vi "MenuButtons.vi"() -> ()   [LabVIEW 2023]
panel:
  in  "ME":bool
  in  "Tacho Interface":bool
  in  "IO Interface":bool
  in  "Datalogger":bool
  in  "Control Station 2":bool
  in  "SF lgi mK1.2 2":bool
  in  "RCS Status":bool
  in  "Cylinder Lubrication":bool
  in  "Shaft Generator":bool
  in  "Axial Vibration":bool
  in  "Hydraulic Power Supply":bool
  in  "Safety System":bool
  in  "Auxiliary System":bool
  in  "Cylinder Configuration":bool
  in  "Turbocharger":bool
  in  "Long Term Test":bool
  in  "Testwall Status":bool
  in  "Report Issue":bool
  in  "Controller Interface":bool
  in  "User Utils":bool
  in  "About":bool
  in  "MOP Parameters":bool
  in  "Update to latest version":bool
  in  "Super Restart Simulation":bool
  in  "MQTT Subscriber":bool
  in  "Show Context Help":bool
  in  "Show Block Diagram":bool
  in  "LabVIEWDev":bool
  in  "Signals On Engine":bool
  in  "Control Station":bool
  in  "Restart Simulation":bool
  in  "Close Screen":bool
  in  "Operate":bool
  # "There's a few of these!"
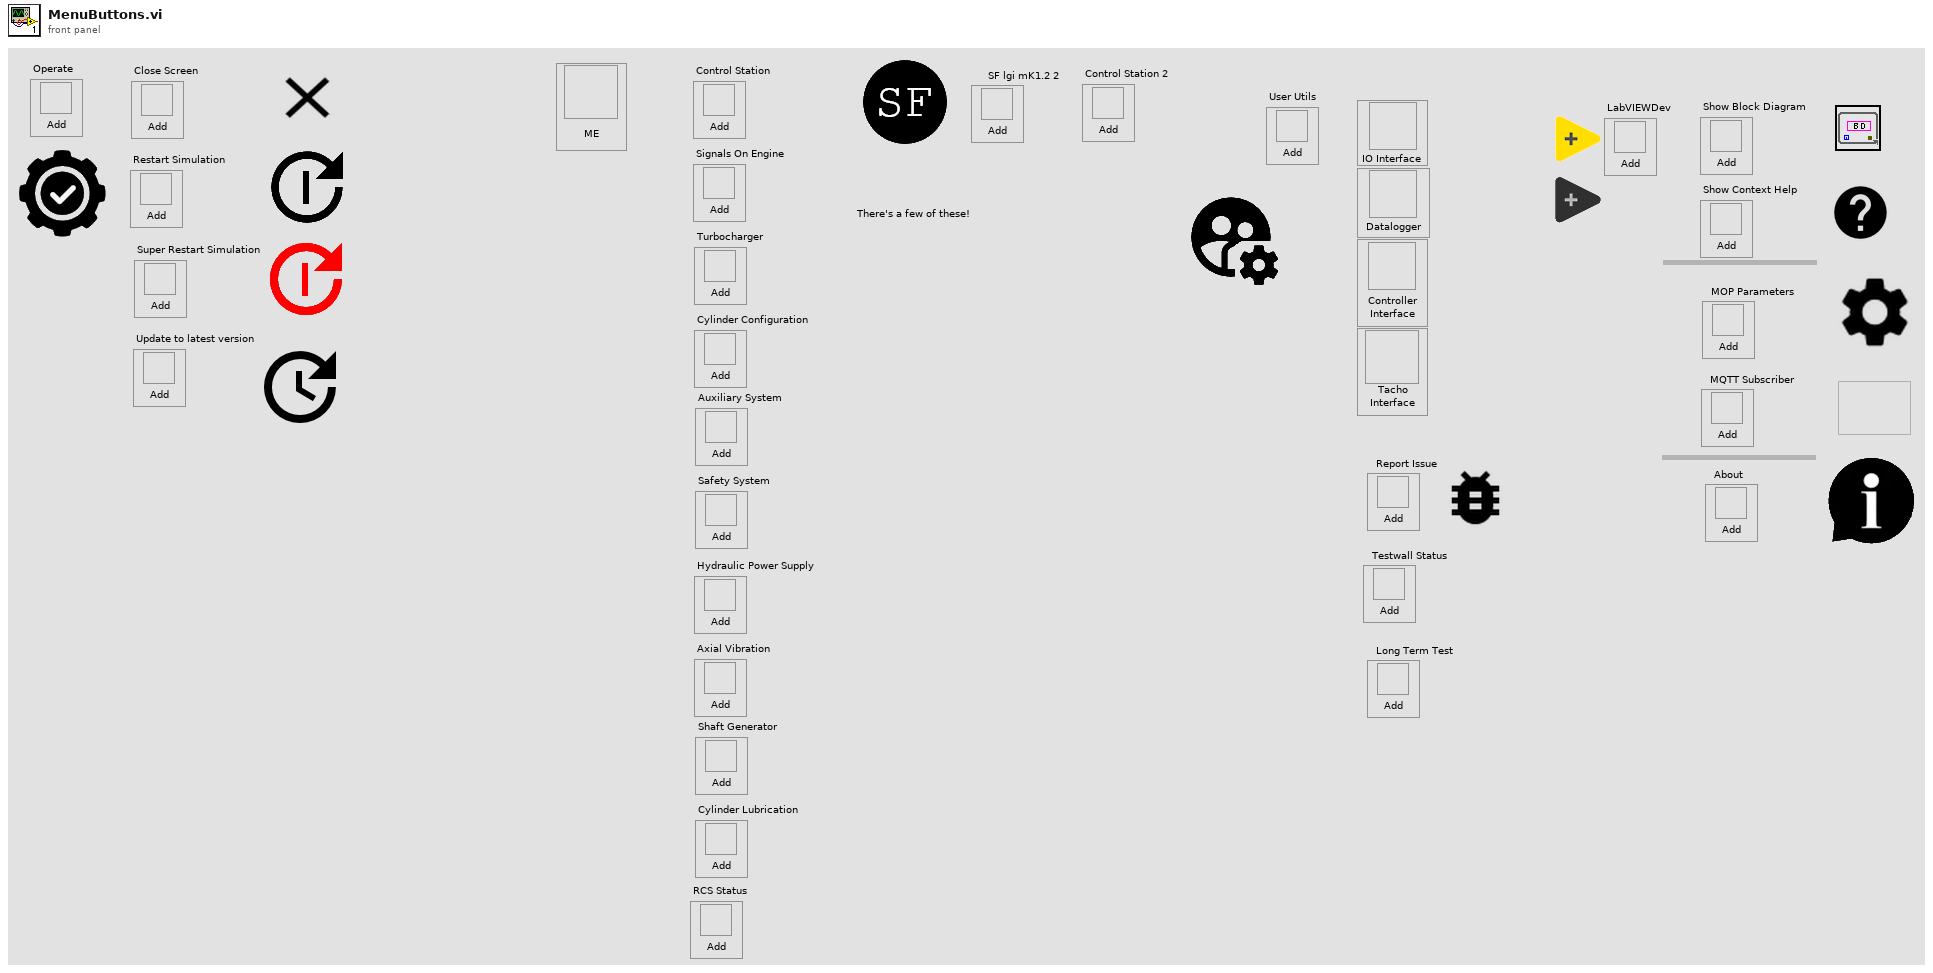
[diagram p1: front panel]
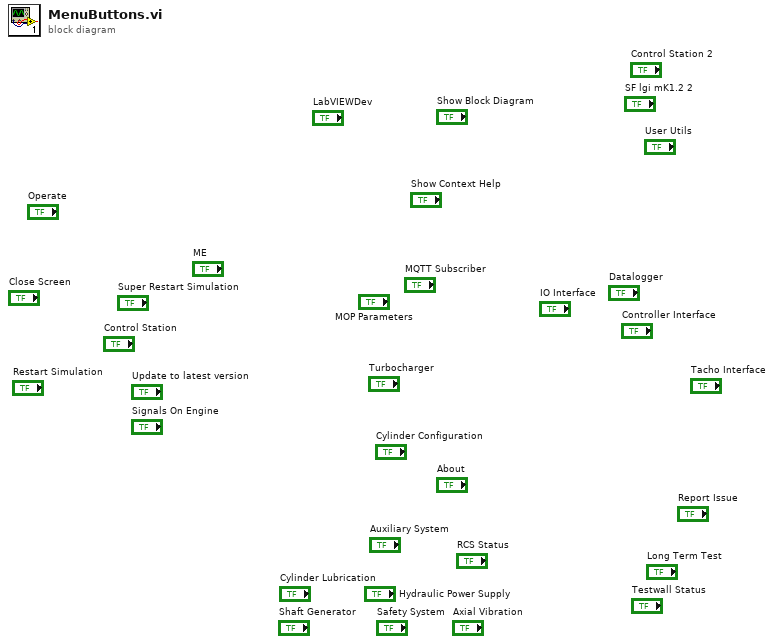
[diagram p0: block diagram]
diagram:
